vi "vi.GlueInternalModule.vi"(8 "error in (no error)":errorcluster, 10 "Data":variant, 11 "Command":string) -> (0 "error out":errorcluster, 3 "Return Data":variant)   [LabVIEW 2014, in "GLue.lvlib" / "class.GLue.lvclass"]
uses:
  class.GLue.lvclass
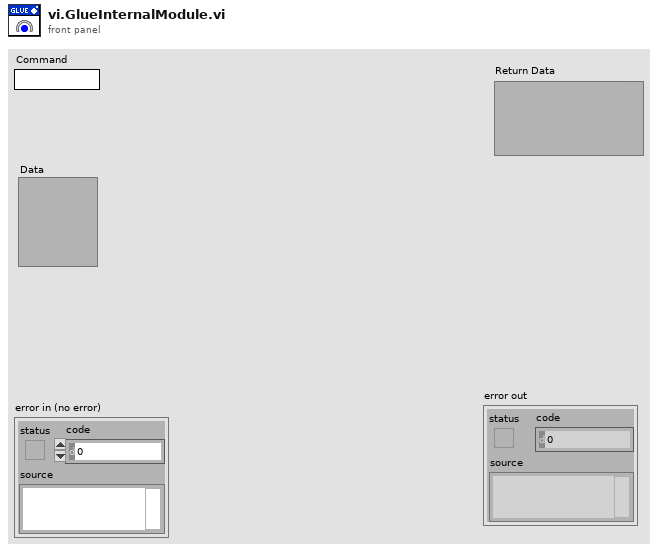
[diagram p1: front panel]
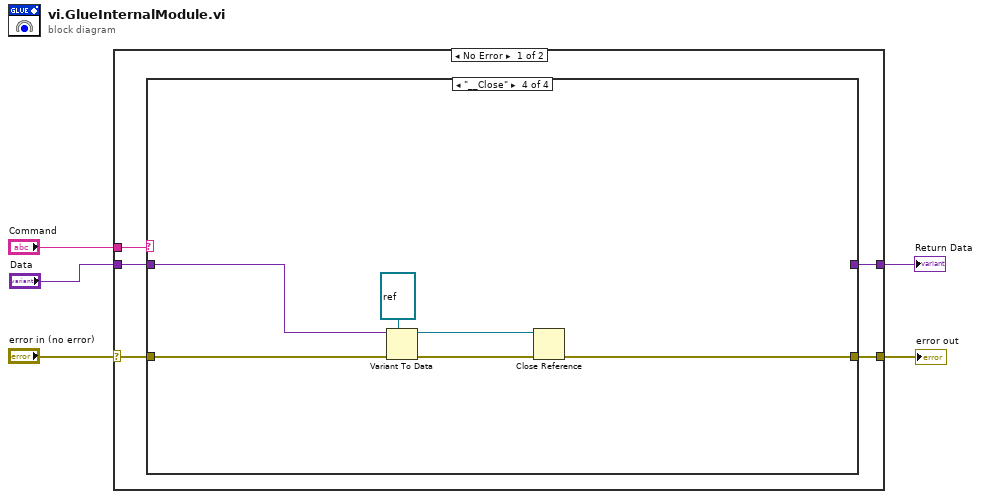
[diagram p0: block diagram]
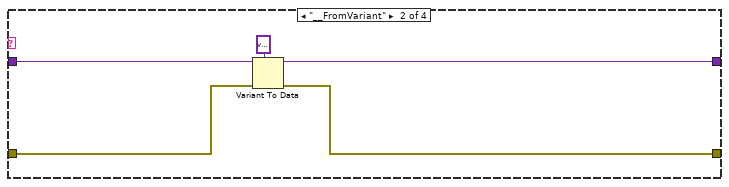
[diagram p3: hidden frame]
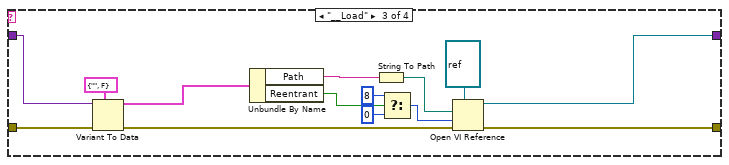
[diagram p4: hidden frame]
diagram:
  n1 = case shown="No Error" "error in (no error)" {
    selector: "error in (no error)" -> [w8 w38]
    tunnel: "Command" -> [w10 _]
    tunnel: "Data" -> [w9 _]
    tunnel: [w7 w38] -> w4
    tunnel: [w6 _] -> w3
    frame No Error {
      n2 = case shown="\"__Close\"" w10 {
        tunnel: w9 -> [w11 w16 w20 w36]
        tunnel: w8 -> [w12 w14 w22 w37]
        tunnel: [w12 w13 w21 w34] -> w7
        tunnel: [w11 w15 w19 _] -> w6
        frame Default {
        }
        frame "__FromVariant" {
          n3 = Variant To Data(error in=w14, type=variant ("Data"), Variant=w16) -> (data=w15:variant, error out=w13:errorcluster)
        }
        frame "__Load" {
          n4 = Variant To Data(error in=w22, type=cluster{"Path":string, "Reentrant":bool} {"Path"="", "Reentrant"=FALSE}, Variant=w20) -> (data=w29:cluster{"Path":string, "Reentrant":bool}, error out=w31:errorcluster)
          n5 = Unbundle By Name(w29) -> ("Path"=w24:string, "Reentrant"=w28:bool)
          n6 = String To Path(string=w24) -> (path=w23:path)
          n7 = Select(t=8 ("options"), s=w28, f=0 ("options")) -> (s? t:f=w26:i32)
          n8 = Open VI Reference(type specifier VI Refnum (for type only)=refnum<vi> refnum, vi path=w23, options=w26, error in (no error)=w31) -> (vi reference=w19:refnum<vi>, error out=w21:errorcluster)  [unwired: 2 in]
        }
        frame "__Close" {
          n9 = Variant To Data(error in=w37, type=refnum<vi> refnum, Variant=w36) -> (data=w33:refnum<vi>, error out=w35:errorcluster)
          n10 = Close Reference(reference=w33, error in (no error)=w35) -> (error out=w34:errorcluster)
        }
      }
    }
    frame Error {
    }
  }
  "Return Data" <- w3
  "error out" <- w4
